vi "ElevatorAtSetpoint.vi"(8 "ElevatorSetpoints":T1=enum."Rest") -> (0 "AtSetpoint":bool)   [LabVIEW 2023]
doc: "Makes sure the actual height of the Elevator is within 0.2 inches of the setpoint/target\n\nAlso tests if wrist is within +/- 3 degrees\n\nInputs:\n--ElevatorSetpoints--Enum\n\nOutputs\n--AtSetpoint--boolean"
uses:
  ElevatorSetpointEnum.ctl
  Wrist/WristGlobal.vi
  ElevatorGlobal.vi
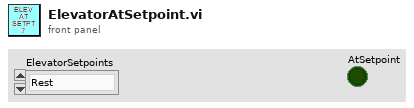
[diagram p1: front panel]
types:
  T1 = typedef "ElevatorSetpointEnum.ctl" = enum16{"Floor", "Rest", "Source", "L1", "L2", "Algae1", "L3", "Algae2", "L4", "Barge", "Processor"}
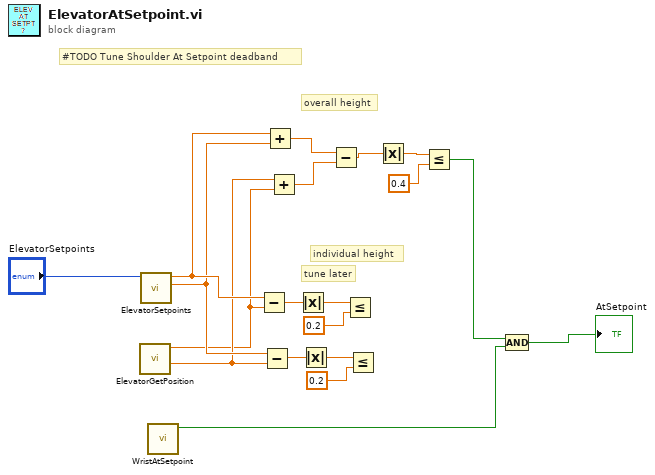
[diagram p0: block diagram]
diagram:
  # "overall height"
  # "individual height"
  # "#TODO Tune Shoulder At Setpoint deadband"
  # "tune later"
  n1 = call "ElevatorGetPosition.vi"() -> ("ElevOuterHeight"=w8:dbl, "ElevStage3Height"=w7:dbl)  [unwired: 9 in, 1 out]
  n2 = call "ElevatorSetpoints.vi"("ElevatorSetpoints"="ElevatorSetpoints") -> ("OuterTargetHeight"=w9:dbl, "Stage3TargetHeight"=w10:dbl)  [unwired: 8 in, 1 out]
  n3 = call "WristAtSetpoint.vi"() -> ("WristAtSetpoint"=w11:bool)  [unwired: 11 in]
  n4 = Subtract(x=w10, y=w7) -> (x-y=w19:dbl)
  n5 = Subtract(x=w9, y=w8) -> (x-y=w15:dbl)
  n6 = Add(x=w10, y=w9) -> (x+y=w6:dbl)
  n7 = Add(x=w8, y=w7) -> (x+y=w5:dbl)
  n8 = Absolute Value(x=w19) -> (abs(x)=w18:dbl)
  n9 = Absolute Value(x=w15) -> (abs(x)=w14:dbl)
  n10 = Subtract(x=w6, y=w5) -> (x-y=w4:dbl)
  n11 = Less Or Equal?(x=w18, y=0.2) -> ()  [unwired: 1 out]
  n12 = Less Or Equal?(x=w14, y=0.2) -> ()  [unwired: 1 out]
  n13 = Absolute Value(x=w4) -> (abs(x)=w3:dbl)
  n14 = Less Or Equal?(x=w3, y=0.4) -> (x <= y?=w1:bool)
  n15 = Compound Arithmetic op=AND(w1, w11) -> (→"AtSetpoint":bool)
